vi "GetDAQtiveChannelNumber.vi"(2 "error in (no error)":errorcluster, 3 "Channel Settings":T1(array[cluster])) -> (0 "error out":errorcluster, 1 "Numeric":i32)   [LabVIEW 2013]
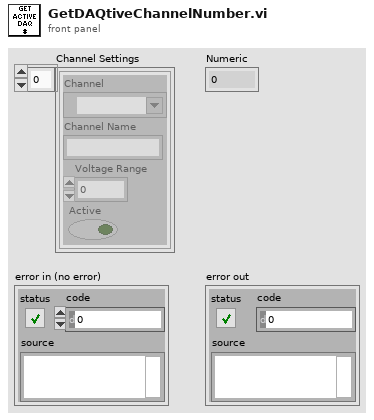
[diagram p1: front panel]
types:
  T1 = cluster{"Channel":tag, "Channel Name":string, "Voltage Range":dbl, "Active":bool}[]
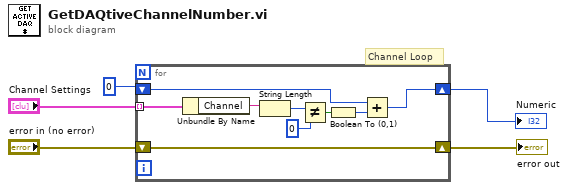
[diagram p0: block diagram]
diagram:
  # "Channel Loop"
  n1 = for {
    tunnel: "Channel Settings" -> [w14] mode=indexing
    shift-right: [w13] -> w2
    shift-left: "error in (no error)" -> [w13]
    shift-right: [w6] -> w5
    shift-left: 0 -> [w7]
    n2 = Unbundle By Name(w14) -> ("Channel"=w12:tag)
    n3 = String Length(string=w12) -> (length=w10:i32)
    n4 = Not Equal?(x=w10, y=0) -> (x != y?=w9:bool)
    n5 = Boolean To (0,1)(Boolean=w9) -> (0, 1=w8:i16)
    n6 = Add(x=w7, y=w8) -> (x+y=w6:i32)
  }
  "Numeric" <- w5
  "error out" <- w2
